vi "Static Error Handling.Parameters.VI Source.Set.vi"(9 "library name (\"\")":string, 10 "vi name":string, 11 "error in":errorcluster) -> (1 "new offset":i32, 3 "error out":errorcluster)   [LabVIEW 2016, in "Static Error Handling.lvlib"]
uses:
  Static Error Handling.lvlib
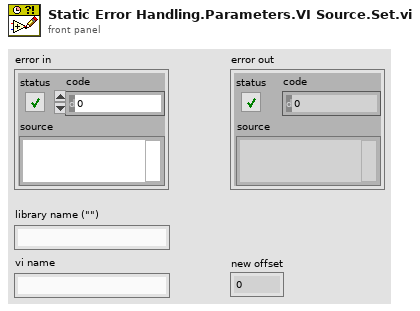
[diagram p1: front panel]
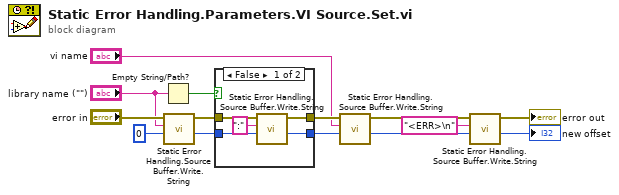
[diagram p0: block diagram]
diagram:
  n1 = Empty String/Path?(string/path="library name (\"\")") -> (empty?=w8:bool)
  n2 = call "Static Error Handling.Source Buffer.Write.String.vi"("offset"=0, "string"="library name (\"\")", "error in"="error in") -> ("new offset"=w6:i32, "error out"=w7:errorcluster)  [unwired: 7 in]
  n3 = case shown="False" w8 {
    tunnel: w7 -> [w19 w21]
    tunnel: w6 -> [w18 w20]
    tunnel: [w17 w21] -> w5
    tunnel: [w16 w20] -> w4
    frame False {
      n4 = call "Static Error Handling.Source Buffer.Write.String.vi"("offset"=w18, "string"=":", "error in"=w19) -> ("new offset"=w16:i32, "error out"=w17:errorcluster)  [unwired: 7 in]
    }
    frame True {
    }
  }
  n5 = call "Static Error Handling.Source Buffer.Write.String.vi"("offset"=w4, "string"="vi name", "error in"=w5) -> ("new offset"=w2:i32, "error out"=w10:errorcluster)  [unwired: 7 in]
  n6 = call "Static Error Handling.Source Buffer.Write.String.vi"("offset"=w2, "string"="<ERR>\n", "error in"=w10) -> ("new offset"=→"new offset":i32, "error out"=→"error out":errorcluster)  [unwired: 7 in]
